vi "Default DB.vi"(8 "error in (no error)":errorcluster) -> (0 "error out":errorcluster, 3 "Data Default":T1)   [LabVIEW 2020, in "COnfiguration Database.lvlib"]
doc: "This VI will return the default Database values."
uses:
  COnfiguration Database.lvlib
  Private Controls/Module Data.ctl
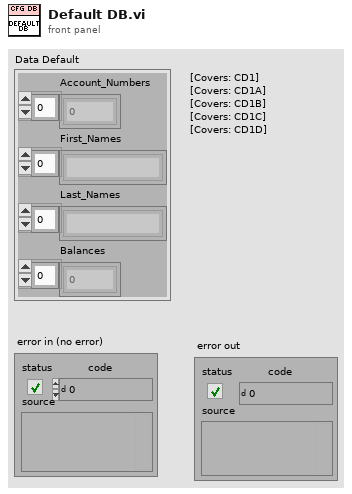
[diagram p1: front panel]
types:
  T1 = typedef "COnfiguration Database.lvlib/Module Data.ctl" = cluster{"Account_Numbers":dbl[], "First_Names":string[], "Last_Names":string[], "Balances":dbl[]}
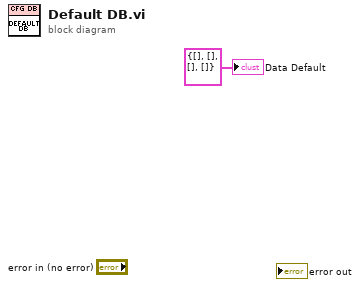
[diagram p0: block diagram]
diagram:
  "Data Default" <- T1 {"Account_Numbers"=[], "First_Names"=[], "Last_Names"=[], "Balances"=[]} ("Data")
